vi "Global_ClimberHWOverride.vi"() -> ()   [LabVIEW 2017, in "Climber.lvlib"]
uses:
  Climber.lvlib
panel:
  in  "Climber Vbus":dbl
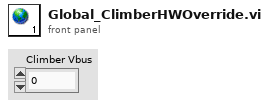
[diagram p1: front panel]
diagram:
